vi "Linear data.vi"(8 "noise amplitude":dbl, 9 "b":dbl, 10 "a":dbl, 11 "Number of points":i32) -> (4 "X Array":i32[](array[numeric]), 5 "Y Array":dbl[](array[numeric]))   [LabVIEW 2023]
doc: "Creates a set of linear data according to the model y = a*x + noise."
uses:
  <vilib>/Analysis/NI_AALBase.lvlib
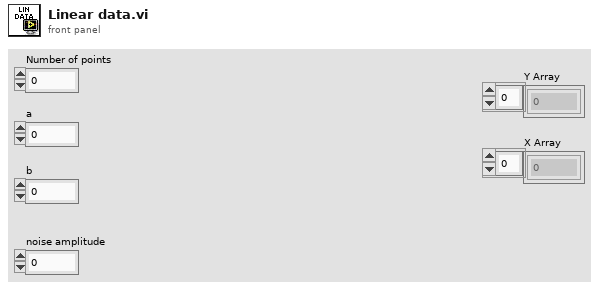
[diagram p1: front panel]
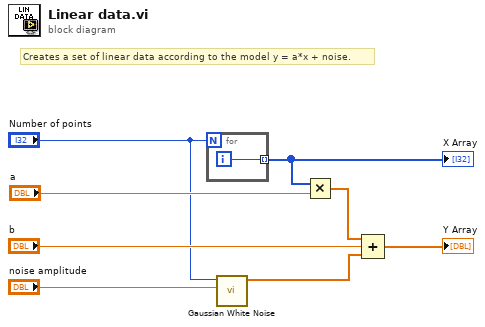
[diagram p0: block diagram]
diagram:
  # "Creates a set of linear data according to the model y = a*x + noise."
  n1 = for {
    N: "Number of points" -> [_]
    tunnel: [w9] -> w8 mode=indexing
    i -> [w9]
  }
  "X Array" <- w8
  n2 = call <vilib>:"Gaussian White Noise.vi"("standard deviation"="noise amplitude", "samples"="Number of points") -> ("Gaussian noise pattern"=w2:dbl[])  [unwired: 8 in, 1 out]
  n3 = Multiply(x=w8, y="a") -> (x*y=w5:dbl[])
  n4 = Compound Arithmetic op=ADD(w5, "b", w2) -> (→"Y Array":dbl[])
